vi "enqueue for data stream.vi"(8 "data":variant, 9 "message":string, 11 "Queues":T1) -> (3 "Queues out":T1)   [LabVIEW 2018]
uses:
  type defs/Queues.ctl
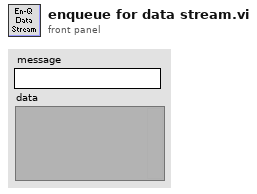
[diagram p1: front panel]
types:
  T1 = typedef "Queues.ctl" = cluster{"messageHandler":refnum<queue>, "comms":refnum<queue>, "dataStream":refnum<queue>, "dataProcessor":refnum<queue>, "fileIO":refnum<queue>, "userInterface":refnum<queue>, "errors":refnum<queue>, "customCompressor":refnum<queue>}
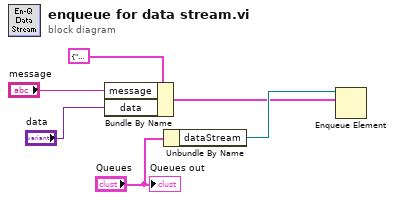
[diagram p0: block diagram]
diagram:
  n1 = Bundle By Name(cluster=cluster{"message":string, "data":variant} {"message"="", "data"=variant} ("element"), "message"="message", "data"="data") -> (w3:cluster{"message":string, "data":variant})
  n2 = Unbundle By Name("Queues") -> ("dataStream"=w5:refnum<queue>)
  n3 = Enqueue Element(queue=w5, element=w3) -> ()  [unwired: 2 in, 3 out]
  "Queues out" <- "Queues"
